vi "Queue Create.vi"(9 "Queue Actor":refnum<class "Queue Actor.lvclass">, 10 "Alias":string, 11 "jettl Queue Actor in":refnum<class "jettl Queue Actor.lvclass">) -> (3 "jettl Queue Actor out":refnum<class "jettl Queue Actor.lvclass">)   [LabVIEW 2021, in "jettl.lvlib" / "jettl Queue Actor.lvclass"]
uses:
  jettl Queue Actor.lvclass
  Actor/Queue Actor/Queue Actor.lvclass
  Actor/Msg/Msg.lvclass
  jettl Queue Actor.lvclass/jettl Queue Actor.ctl
  jettl.lvlib
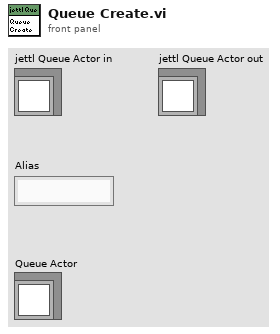
[diagram p1: front panel]
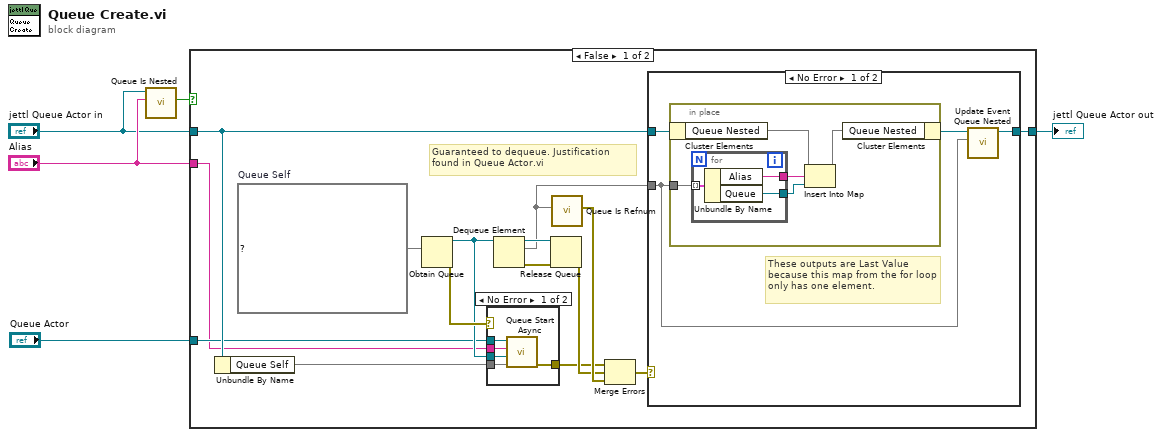
[diagram p0: block diagram]
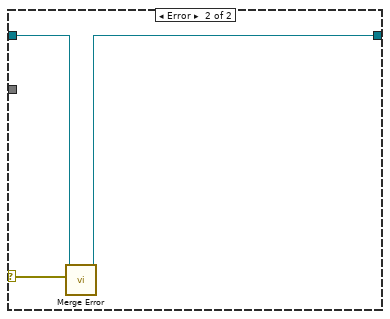
[diagram p3: hidden frame]
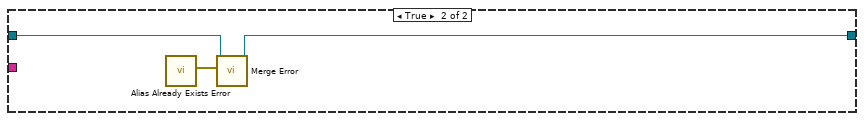
[diagram p4: hidden frame]
diagram:
  n1 = call-dynamic "Queue Is Nested.vi"("Alias"="Alias", "jettl Queue Actor in"="jettl Queue Actor in") -> ("Queue Is Nested?"=w3:bool)  [unwired: 9 in]
  n2 = case shown="False" w3 {
    tunnel: "Queue Actor" -> [w8 _]
    tunnel: "jettl Queue Actor in" -> [w15 w44]
    tunnel: "Alias" -> [w6 _]
    tunnel: [w14 w43] -> w4
    frame False {
      w10 = map{string, refnum<data-value>} {}  # Queue Self
      # "Guaranteed to dequeue. Justification found in Queue Actor.vi"
      n3 = Unbundle By Name(w15) -> ("Queue Self"=w16:map{string, refnum<data-value>})
      n4 = Obtain Queue(element data type=w10) -> (queue out=w9:refnum<queue>, error out=w20:errorcluster)  [unwired: 4 in, 1 out]
      n5 = case shown="No Error" w20 {
        selector: w20 -> [_ w26]
        tunnel: [w24 w26] -> w11
        tunnel: w8 -> [w25 _]
        tunnel: w16 -> [w22 _]
        tunnel: w9 -> [w23 _]
        tunnel: w6 -> [w21 _]
        frame No Error {
          n6 = call "Queue Start Async.vi"("Queue Caller"=w22, "Queue of Queue Self"=w23, "Queue Self Alias"=w21, "Queue Actor"=w25) -> ("error out"=w24:errorcluster)  [unwired: 7 in]
        }
        frame Error {
        }
      }
      n7 = Dequeue Element(queue=w9) -> (queue out=w18:refnum<queue>, element=w7:map{string, refnum<data-value>}, error out=w19:errorcluster)  [unwired: 2 in, 1 out]
      n8 = Release Queue(queue=w18, error in (no error)=w19) -> (error out=w12:errorcluster)  [unwired: 1 in, 2 out]
      n9 = call "Queue Is Refnum.vi"("Queue Self"=w7) -> ("Error"=w13:errorcluster)  [unwired: 10 in]
      n10 = Merge Errors(w11, w12, w13) -> (w17:errorcluster)
      n11 = case shown="No Error" w17 {
        selector: w17 -> [_ w39]
        tunnel: w15 -> [w30 w41]
        tunnel: [w28 w40] -> w14
        tunnel: w7 -> [w27 _]
        frame No Error {
          # "These outputs are Last Value because this map from the for loop only has one element."
          n12 = in-place {
            in-place-border: w27 -> [w33]
            n13 = in-place-cluster #1(w30) -> ("Queue Nested"=w35:map{string, refnum<data-value>})
            n14 = for {
              tunnel: w33 -> [w38] mode=indexing
              tunnel: [w37] -> w32
              tunnel: [w36] -> w31
              n15 = Unbundle By Name(w38) -> ("Alias"=w37:string, "Queue"=w36:refnum<data-value>)
            }
            n16 = Insert Into Map(map in=w35, key=w32, value=w31) -> (map out=w34:map{string, refnum<data-value>})  [unwired: 2 out]
            n17 = in-place-cluster #1("Queue Nested"=w34) -> (w29:refnum<class "jettl Queue Actor.lvclass">)
          }
          n18 = call "Update Event Queue Nested.vi"("Queue Nested"=w27, "jettl Queue Actor in"=w29) -> ("jettl Queue Actor out"=w28:refnum<class "jettl Queue Actor.lvclass">)  [unwired: 9 in]
        }
        frame Error {
          n19 = call-dynamic "Merge Error.vi"("Error"=w39, "jettl Queue Actor in"=w41) -> ("jettl Queue Actor out"=w40:refnum<class "jettl Queue Actor.lvclass">)  [unwired: 9 in]
        }
      }
    }
    frame True {
      n20 = call "Alias Already Exists Error.vi"() -> ("Error"=w42:errorcluster)  [unwired: 11 in]
      n21 = call-dynamic "Merge Error.vi"("Error"=w42, "jettl Queue Actor in"=w44) -> ("jettl Queue Actor out"=w43:refnum<class "jettl Queue Actor.lvclass">)  [unwired: 9 in]
    }
  }
  "jettl Queue Actor out" <- w4
